vi "SQL_Insert.vi"(7 "表名":string, 8 "error in (no error)":errorcluster, 9 "值":string[](array[string]), 10 "列名":string[](array[string]), 11 "connection reference":T1) -> (0 "error out":errorcluster, 3 "connection reference 2":T1)   [LabVIEW 2018]
uses:
  <vilib>/addons/database/Connection.llb/Conn ObjectReference.ctl
  <vilib>/addons/database/Connection.llb/Conn Execute.vi
  <vilib>/addons/database/Recordset.llb/Rec Destroy - Connection.vi
  <vilib>/addons/database/NI_Database_API.lvlib
panel:
  out "连接的字符串":string
  # "语法："
  # "INSERT INTO 表名称 VALUES (值1, 值2,....)"
  # "INSERT INTO table_name (列1, 列2,...) VALUES (值1, 值2,....)"
  # "若插入为整行时可不填"
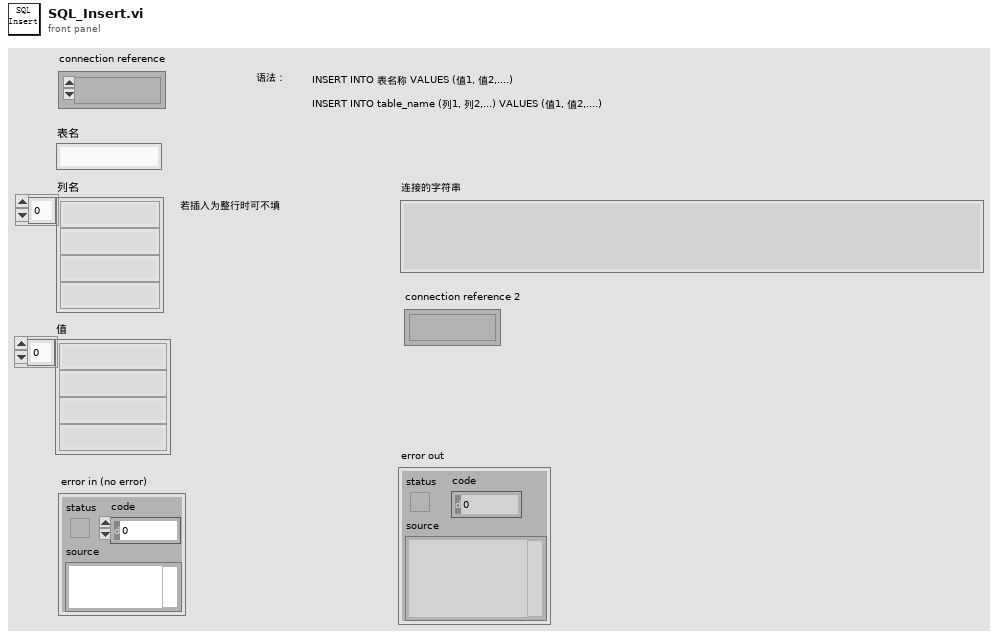
[diagram p1: front panel]
types:
  T1 = typedef "NI_Database_API.lvlib/Conn ObjectReference.ctl" = refnum<k1>
  T2 = typedef "NI_Database_API.lvlib/Rec ObjectReference.ctl" = refnum<k1>
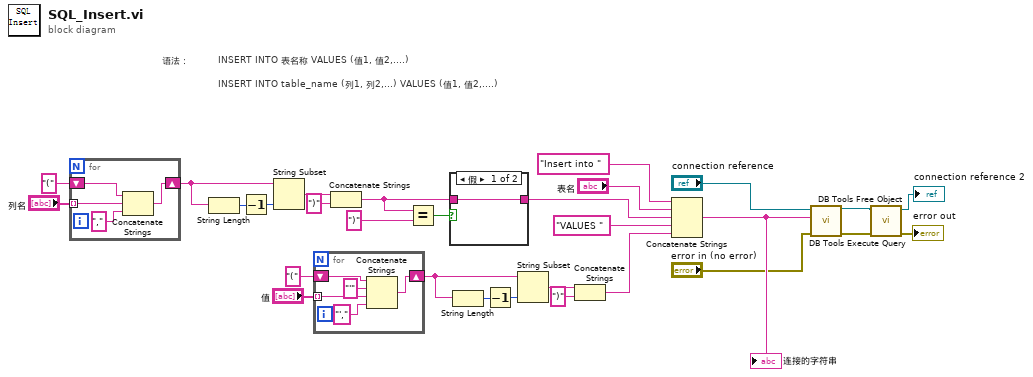
[diagram p0: block diagram]
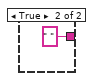
[diagram p2: hidden frame]
diagram:
  # "语法："
  # "INSERT INTO table_name (列1, 列2,...) VALUES (值1, 值2,....)"
  # "INSERT INTO 表名称 VALUES (值1, 值2,....)"
  n1 = for {
    tunnel: "列名" -> [w33] mode=indexing
    shift-right: [w32] -> w21
    shift-left: "(" -> [w30]
    n2 = Concatenate Strings(w30, w33, "," ("字符串")) -> (w32:string)
  }
  n3 = String Length(string=w21) -> (length=w20:i32)
  n4 = Decrement(x=w20) -> (x-1=w19:i32)
  n5 = String Subset(string=w21, length (rest)=w19) -> (substring=w18:string)  [unwired: 1 in]
  n6 = for {
    tunnel: "值" -> [w38] mode=indexing
    shift-right: [w37] -> w11
    shift-left: "(" -> [w35]
    n7 = Concatenate Strings(w35, "'" ("字符串"), w38, "'," ("字符串")) -> (w37:string)
  }
  n8 = Concatenate Strings(w18, ")" ("字符串")) -> (w5:string)
  n9 = Equal?(x=w5, y=")") -> (x = y?=w6:bool)
  n10 = case shown="假" w6 {
    tunnel: w5 -> [w39 _]
    tunnel: [w39 " "] -> w4
    frame False {
    }
    frame True {
    }
  }
  n11 = String Length(string=w11) -> (length=w12:i32)
  n12 = Decrement(x=w12) -> (x-1=w13:i32)
  n13 = String Subset(string=w11, length (rest)=w13) -> (substring=w14:string)  [unwired: 1 in]
  n14 = Concatenate Strings(w14, ")" ("字符串")) -> (w8:string)
  n15 = Concatenate Strings("Insert into ", "表名", w4, "VALUES " ("字符串"), w8) -> (w26:string)
  "连接的字符串" <- w26
  n16 = call-poly <vilib>:"DB Tools Execute Query.vi"("error in (no error)"="error in (no error)", "SQL query"=w26, "connection reference"="connection reference") -> ("error out"=w2:errorcluster, "recordset reference"=w3:T2)  [unwired: 5 in]
  n17 = call-poly <vilib>:"DB Tools Free Object.vi"("error in (no error)"=w2, "recordset reference"=w3) -> ("error out"=→"error out":errorcluster, "connection reference"=→"connection reference 2":T1)  [unwired: 8 in]
